vi "Read Server Hostname.vi"(8 "error in (no error)":errorcluster, 11 "SSL Client Socket in":refnum<class "SSL Client Socket.lvclass">) -> (0 "error out":errorcluster, 2 "Server Hostname":string, 3 "SSL Client Socket out":refnum<class "SSL Client Socket.lvclass">)   [LabVIEW 2013, in "OpenSSL Socket.lvlib" / "SSL Client Socket.lvclass"]
uses:
  SSL Client Socket.lvclass
  SSL Client Socket.lvclass/SSL Client Socket.ctl
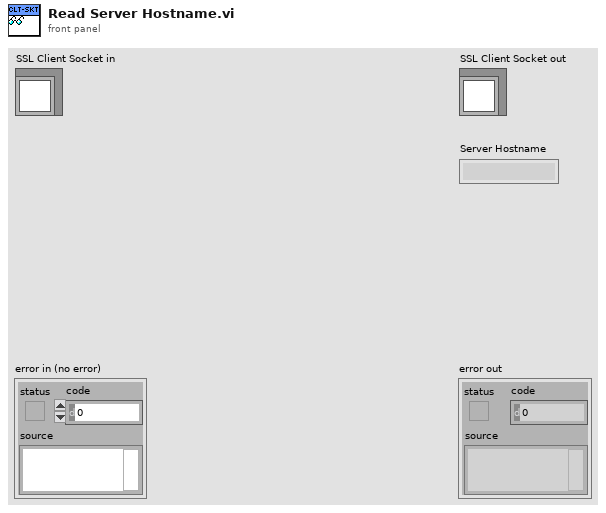
[diagram p1: front panel]
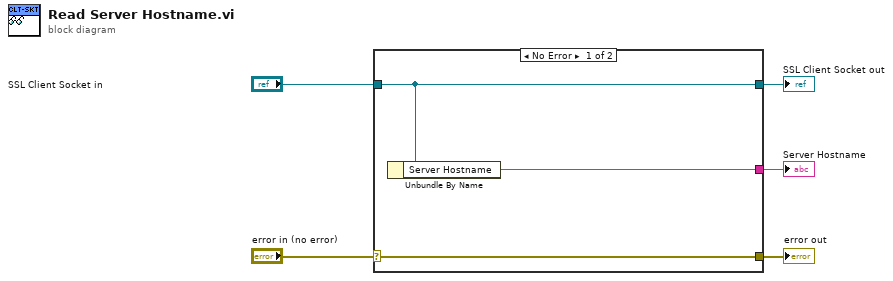
[diagram p0: block diagram]
diagram:
  n1 = case shown="No Error" "error in (no error)" {
    selector: "error in (no error)" -> [w8 w9]
    tunnel: [w8 w9] -> w4
    tunnel: [w7 w10] -> w2
    tunnel: "SSL Client Socket in" -> [w7 w10]
    tunnel: [w6 _] -> w1
    frame No Error {
      n2 = Unbundle By Name(w7) -> ("Server Hostname"=w6:string)
    }
    frame Error {
    }
  }
  "error out" <- w4
  "SSL Client Socket out" <- w2
  "Server Hostname" <- w1
